vi "Potenciometro.vi"(8 "error in (no error)":errorcluster, 9 "Wavelength (0.0)":dbl, 11 "num Lect":i32) -> (0 "error out":errorcluster, 1 "Valor Actual":dbl, 2 "Valor Prom":dbl)   [LabVIEW 2018]
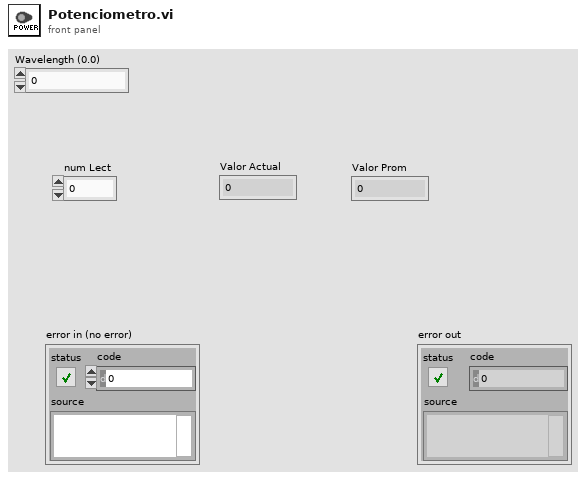
[diagram p1: front panel]
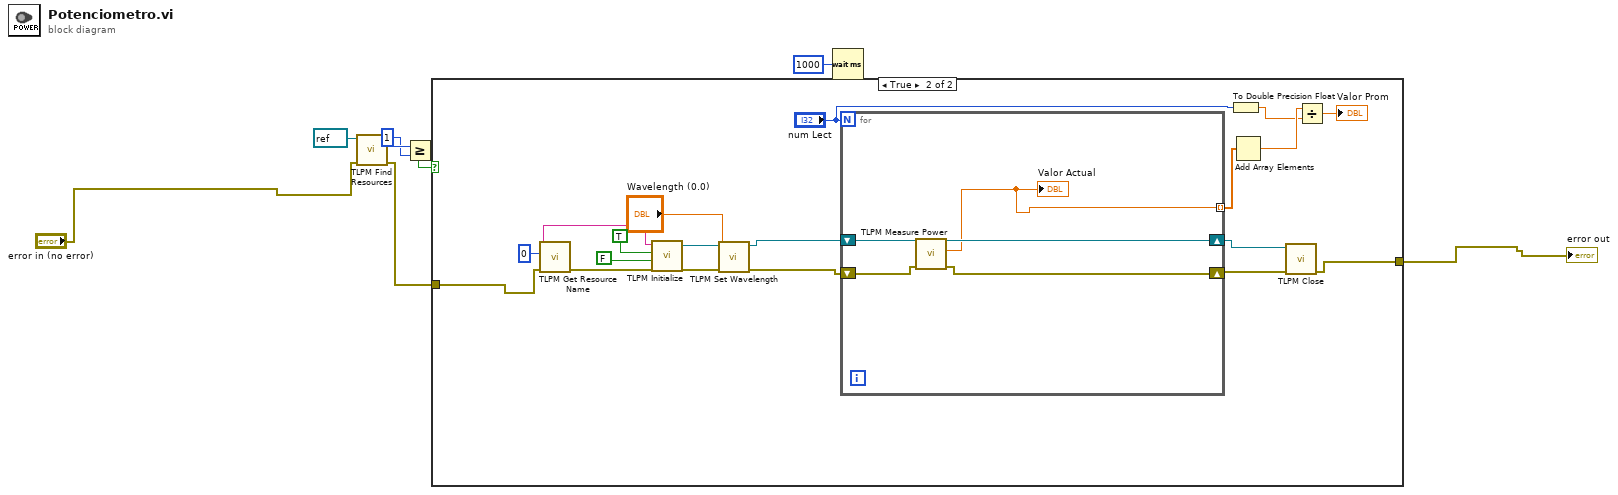
[diagram p0: block diagram]
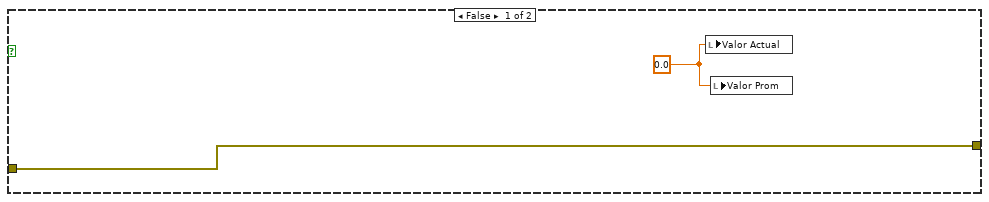
[diagram p2: hidden frame]
diagram:
  n1 = call <instrlib>:"TLPM Find Resources.vi"("error in (no error)"="error in (no error)", "instrument handle"=refnum<visa-resource-name> refnum) -> ("error out"=w3:errorcluster, "Resource Count"=w7:u32)  [unwired: 7 in, 1 out]
  n2 = Greater Or Equal?(x=w7, y=u32 1) -> (x >= y?=w4:bool)
  n3 = case shown="True" w4 {
    tunnel: [w9 w17] -> w2
    tunnel: w3 -> [w9 w16]
    frame False {
      w10 = 0.0
      n4 = local write "Valor Actual"(w10) -> ()
      n5 = local write "Valor Prom"(w10) -> ()
    }
    frame True {
      n6 = call <instrlib>:"TLPM Get Resource Name.vi"("error in (no error)"=w16, "Index (0)"=u32 0 ("Device Index")) -> ("error out"=w29:errorcluster, "Resource Name"=w28:string)  [unwired: 7 in, 1 out]
      n7 = call <instrlib>:"TLPM Initialize.vi"("error in (no error)"=w29, "Reset Device (Reset Device)"=FALSE ("ID Query (Do Query)"), "ID Query (Do Query)"=TRUE, "resource name"=w28) -> ("error out"=w13:errorcluster, "instrument handle out"=w15:refnum<visa-resource-name>)  [unwired: 6 in]
      n8 = call <instrlib>:"TLPM Set Wavelength.vi"("error in (no error)"=w13, "Wavelength (0.0)"="Wavelength (0.0)", "instrument handle"=w15) -> ("error out"=w11:errorcluster, "instrument handle out"=w12:refnum<visa-resource-name>)  [unwired: 7 in]
      n9 = for {
        N: "num Lect" -> [_]
        shift-right: [w32] -> w18
        shift-left: w11 -> [w33]
        shift-right: [w31] -> w19
        shift-left: w12 -> [w34]
        tunnel: [w30] -> w24 mode=indexing
        n10 = call <instrlib>:"TLPM Measure Power.vi"("error in (no error)"=w33, "instrument handle"=w34) -> ("error out"=w32:errorcluster, "Power"=w30:dbl, "instrument handle out"=w31:refnum<visa-resource-name>)  [unwired: 7 in]
        "Valor Actual" <- w30
      }
      n11 = To Double Precision Float(number="num Lect") -> (double precision float=w20:dbl)
      n12 = Add Array Elements(numeric array=w24) -> (sum=w22:dbl)
      n13 = call <instrlib>:"TLPM Close.vi"("error in (no error)"=w18, "instrument handle"=w19) -> ("error out"=w17:errorcluster)  [unwired: 9 in]
      n14 = Divide(x=w22, y=w20) -> (x/y=→"Valor Prom":dbl)
    }
  }
  "error out" <- w2
  n15 = Wait (ms)(milliseconds to wait=u32 1000) -> ()  [unwired: 1 out]
